vi "Read.Initialize.vi"(8 "error in (no error)":errorcluster, 11 "Read in":refnum<class "Read.lvclass">) -> (0 "error out":errorcluster, 3 "Read out":refnum<class "Read.lvclass">)   [LabVIEW 2015, in "Data Access API.lvlib" / "Read.lvclass"]
uses:
  Read.lvclass
  Read.lvclass/Read.ctl
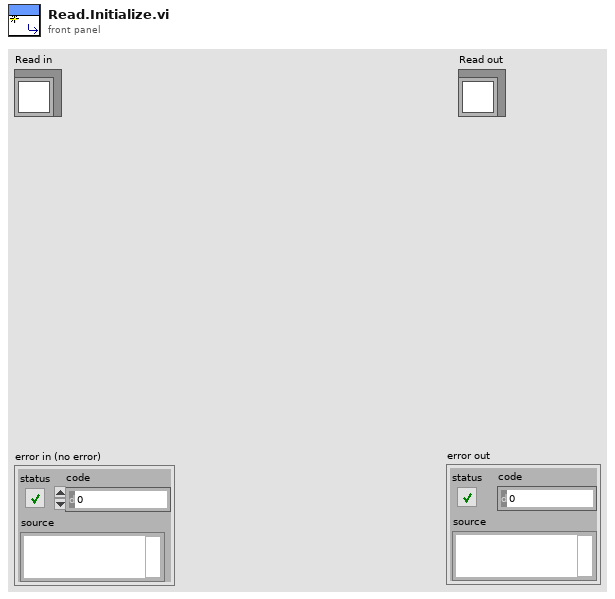
[diagram p1: front panel]
types:
  T1 = cluster{"read mode":enum16{"polling", "blocking"}, "write mode":enum16{"polling", "blocking"}}
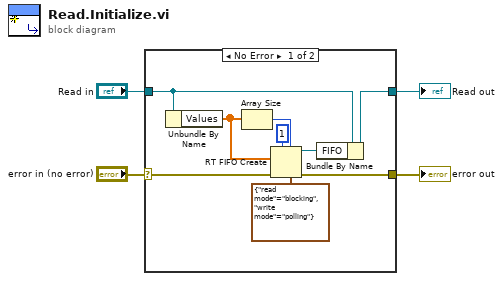
[diagram p0: block diagram]
diagram:
  n1 = case shown="No Error" "error in (no error)" {
    selector: "error in (no error)" -> [w5 w15]
    tunnel: [w11 w15] -> w4
    tunnel: "Read in" -> [w7 w14]
    tunnel: [w6 w14] -> w2
    frame No Error {
      n2 = Unbundle By Name(w7) -> ("Values"=w8:dbl[])
      n3 = Array Size(array=w8) -> (size(s)=w10:i32)
      n4 = RT FIFO Create(1:w8, 3:w5, 4:u32 1 ("size (10)"), 6:w10, 7:T1 {"read mode"=enum."blocking", "write mode"=enum."polling"} ("r/w modes (polling,polling)")) -> (8:w13:refnum<k33>, 11:w11:errorcluster)  [unwired: 3 in, 1 out]
      n5 = Bundle By Name(cluster=w7, "FIFO"=w13) -> (w6:refnum<class "Read.lvclass">)
    }
    frame Error {
    }
  }
  "error out" <- w4
  "Read out" <- w2
